vi "Do.vi"(8 "error in (no error)":errorcluster, 10 "Actor in":refnum<class "Actor.lvclass">, 11 "Update Meta data Msg":refnum<class "Update Meta data Msg.lvclass">) -> (0 "error out":errorcluster, 2 "Actor out":refnum<class "Actor.lvclass">)   [LabVIEW 2018, in "TCP Classes.lvlib" / "Update Meta data Msg.lvclass"]
doc: "This VI delivers the message to the actor by calling the appropriate method(s) on the actor."
uses:
  Update Meta data Msg.lvclass
  <vilib>/ActorFramework/Actor/Actor.lvclass
  Class TCP Connection/TCP Connection.lvclass
  C:/Program Files (x86)/National Instruments/LabVIEW 2018/vi.lib/ActorFramework/Actor/Actor.lvclass
  Update Meta data Msg.lvclass/Update Meta data Msg.ctl
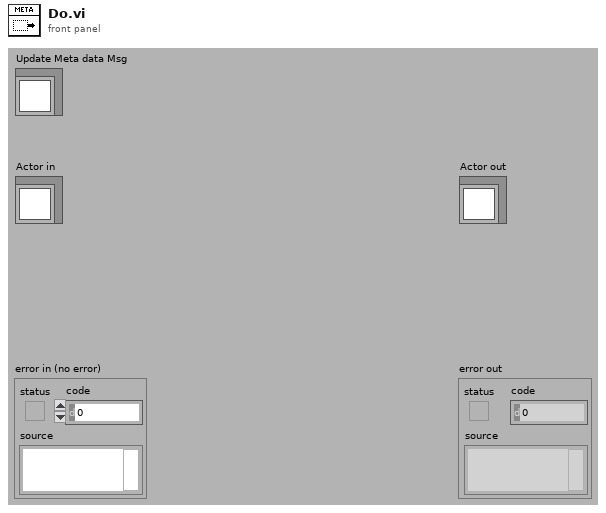
[diagram p1: front panel]
types:
  T1 = typedef "stm_MetaDataElement.ctl" = string
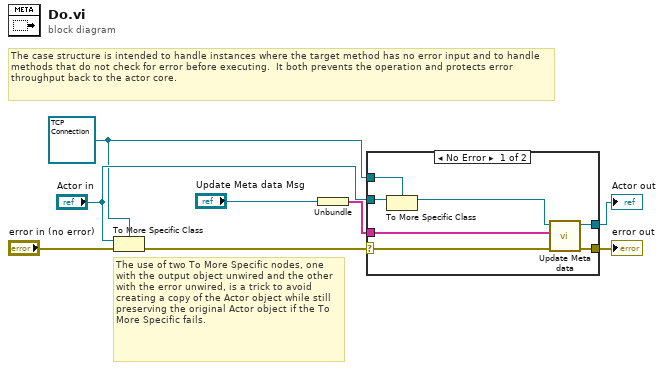
[diagram p0: block diagram]
diagram:
  w2 = refnum<class "TCP Connection.lvclass"> refnum ("Actor in")
  # "The use of two To More Specific nodes, one with the output object unwired and the other with the error unwired, is a trick to avoid creating a copy of the Actor object while still preserving the original Actor object if the To More Specific fails."
  # "The case structure is intended to handle instances where the target method has no error input and to handle methods that do not check for error before executing.  It both prevents the operation and protects error throughput back to the actor core."
  n1 = To More Specific Class(target class=w2, reference="Actor in", error in="error in (no error)") -> (error out=w6:errorcluster)  [unwired: 1 out]
  n2 = Unbundle("Update Meta data Msg") -> (w1:T1[])
  n3 = case shown="No Error" w6 {
    selector: w6 -> [w13 w17]
    tunnel: [w15 w17] -> w5
    tunnel: [w14 w16] -> w4
    tunnel: "Actor in" -> [w12 w16]
    tunnel: w2 -> [w11 _]
    tunnel: w1 -> [w9 _]
    frame No Error {
      n4 = To More Specific Class(target class=w11, reference=w12) -> (specific class reference=w10:refnum<class "TCP Connection.lvclass">)  [unwired: 1 in, 1 out]
      n5 = call "Update Meta data.vi"("error in (no error)"=w13, "Meta data"=w9, "TCP Connection in"=w10) -> ("error out"=w15:errorcluster, "TCP Connection out"=w14:refnum<class "TCP Connection.lvclass">)  [unwired: 7 in]
    }
    frame Error {
      # "If type check fails, pass the original object out again."
    }
  }
  "error out" <- w5
  "Actor out" <- w4
